vi "New Configuration Error.vi"(7 "error source vi name":string, 11 "configuration error":T1) -> (1 "new offset":i32, 3 "error out":errorcluster)   [LabVIEW 2017, in "DSF Core.lvlib" / "Configuration Session.lvclass"]
uses:
  Configuration Session.lvclass
  Errors.ctl
  VIs/Constants/Engine Library Name.vi
  <vilib>/NI/Memory Manager/VIs/New Error Cluster (512B).vi
  <vilib>/NI/Memory Manager/Static Errors.lvlib
  Framework/Framework.lvclass
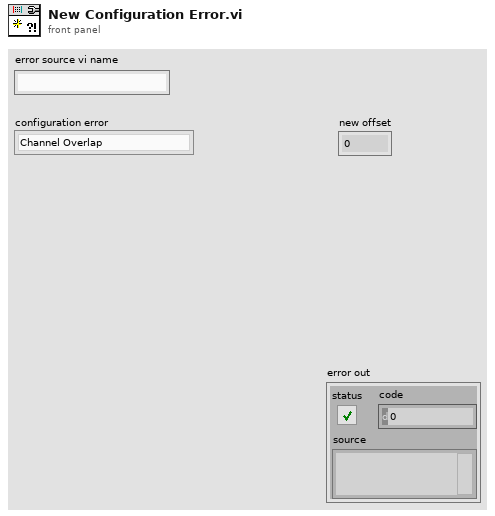
[diagram p1: front panel]
types:
  T1 = typedef "DSF Core.lvlib/Configuration Session.lvclass/Errors.ctl" = enum16{"Channel Overlap", "Invalid Engine Offset", "Invalid JSON"}
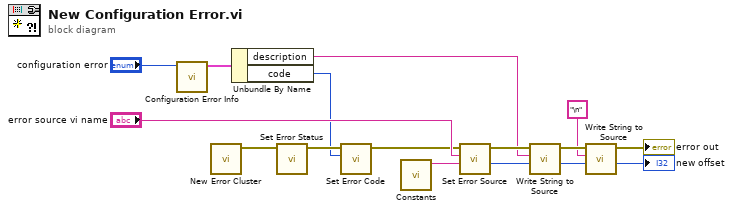
[diagram p0: block diagram]
diagram:
  n1 = call "Configuration Error Info.vi"("configuration error"="configuration error") -> ("error info"=w8:cluster{"code":i32, "description":string})  [unwired: 10 in]
  n2 = call-poly <vilib>:"New Error Cluster.vi"() -> ("error out"=w14:errorcluster)  [unwired: 10 in, 1 out]
  n3 = Unbundle By Name(w8) -> ("description"=w6:string, "code"=w7:i32)
  n4 = call <vilib>:"Set Error Status.vi"("error in"=w14) -> ("error out"=w13:errorcluster)  [unwired: 9 in, 1 out]
  n5 = call <vilib>:"Set Error Code.vi"("code"=w7, "error in"=w13) -> ("error out"=w12:errorcluster)  [unwired: 8 in, 1 out]
  n6 = call-poly "Constants.vi"() -> ("Engine Library Name"=w10:string)  [unwired: 11 in]
  n7 = call <vilib>:"Set Error Source.vi"("library name (\"\")"=w10, "vi name"="error source vi name", "error in"=w12) -> ("initial offset"=w9:i32, "error out"=w11:errorcluster)  [unwired: 7 in]
  n8 = call <vilib>:"Write String to Source.vi"("offset"=w9, "string"=w6, "error in"=w11) -> ("new offset"=w2:i32, "error out"=w5:errorcluster)  [unwired: 7 in]
  n9 = call <vilib>:"Write String to Source.vi"("offset"=w2, "string"="\n", "error in"=w5) -> ("new offset"=→"new offset":i32, "error out"=→"error out":errorcluster)  [unwired: 7 in]
